vi "classes array.vi"() -> (0 "MBs":refnum<class "Master CR.lvclass">[](array[class]))   [LabVIEW 2021, in "Master CR.lvclass"]
uses:
  Master CR.lvclass
  Devices/M7000/ICPCON PM-3112 RTU/ICPCON PM-3112-RTU.lvclass
  D:/my_projects/projects/Algorithms/Labview/21/Master CR/Master CR.lvclass
  Devices/ET7000/ICPCON ET-7017/ICPCON ET-7017.lvclass
  Devices/ET7000/ICPCON PM-3112/ICPCON PM-3112.lvclass
  Devices/ET7000/ICPCON ET-7051/ICPCON ET-7051.lvclass
  Devices/ET7000/ICPCON ET-7042/ICPCON ET-7042.lvclass
  Devices/ET7000/ICPCON ET-7028/ICPCON ET-7028.lvclass
  Devices/ET7000/ICPCON ET-7024/ICPCON ET-7024.lvclass
  Devices/ET7000/ICPCON ET-7018/ICPCON ET-7018.lvclass
  Devices/ET7000/ICPCON ET-7018i/ICPCON ET-7018i.lvclass
  Devices/ET7000/ICPCON ET-7017-10/ICPCON ET-7017-10.lvclass
  Devices/SMSD/SMSD-DI/SMSD-DI.lvclass
  Devices/SMSD/SMSD-AI/SMSD-AI.lvclass
  Devices/M7000/ICPCON M-7024/ICPCON M-7024.lvclass
  Devices/Serial/ELAN/ELAN.lvclass
  Devices/ET7000/TEST1/TEST1.lvclass
  Devices/ET7000/TEST/TEST.lvclass
  Devices/ET7000/ICPCON ET-7016i/ICPCON ET-7016i.lvclass
  Master CR.lvclass/Master CR.ctl
  Devices/ET7000/ICPCON ET-7042UR/ICPCON ET-7042UR.lvclass
  D:/my_projects/projects/Algorithms/Labview/21/Master CR/Devices/ET7000/TCP/TCP.lvclass
  D:/my_projects/projects/Algorithms/Labview/21/Master CR/Devices/ET7000/TEST/TEST.lvclass
  D:/my_projects/projects/Algorithms/Labview/21/Master CR/Devices/ET7000/TEST1/TEST1.lvclass
  D:/my_projects/projects/Algorithms/Labview/21/Master CR/Devices/ET7000/ICPCON ET-7016i/ICPCON ET-7016i.lvclass
  D:/my_projects/projects/Algorithms/Labview/21/Master CR/Devices/ET7000/ICPCON ET-7017/ICPCON ET-7017.lvclass
  D:/my_projects/projects/Algorithms/Labview/21/Master CR/Devices/ET7000/ICPCON ET-7017-10/ICPCON ET-7017-10.lvclass
  D:/my_projects/projects/Algorithms/Labview/21/Master CR/Devices/ET7000/ICPCON ET-7018i/ICPCON ET-7018i.lvclass
  D:/my_projects/projects/Algorithms/Labview/21/Master CR/Devices/ET7000/ICPCON ET-7018/ICPCON ET-7018.lvclass
  D:/my_projects/projects/Algorithms/Labview/21/Master CR/Devices/ET7000/ICPCON ET-7024/ICPCON ET-7024.lvclass
  D:/my_projects/projects/Algorithms/Labview/21/Master CR/Devices/ET7000/ICPCON ET-7028/ICPCON ET-7028.lvclass
  D:/my_projects/projects/Algorithms/Labview/21/Master CR/Devices/ET7000/ICPCON ET-7042/ICPCON ET-7042.lvclass
  D:/my_projects/projects/Algorithms/Labview/21/Master CR/Devices/ET7000/ICPCON ET-7042UR/ICPCON ET-7042UR.lvclass
  D:/my_projects/projects/Algorithms/Labview/21/Master CR/Devices/ET7000/ICPCON ET-7051/ICPCON ET-7051.lvclass
  D:/my_projects/projects/Algorithms/Labview/21/Master CR/Devices/ET7000/ICPCON PM-3112/ICPCON PM-3112.lvclass
  D:/my_projects/projects/Algorithms/Labview/21/Master CR/Devices/Serial/Modbus Serial/Modbus Serial.lvclass
  D:/my_projects/projects/Algorithms/Labview/21/Master CR/Devices/Serial/Serial.lvclass
  D:/my_projects/projects/Algorithms/Labview/21/Master CR/Devices/M7000/ICPCON M-7024/ICPCON M-7024.lvclass
  D:/my_projects/projects/Algorithms/Labview/21/Master CR/Devices/M7000/ICPCON PM-3112 RTU/ICPCON PM-3112-RTU.lvclass
  D:/my_projects/projects/Algorithms/Labview/21/Master CR/Devices/Serial/ELAN/ELAN.lvclass
  D:/my_projects/projects/Algorithms/Labview/21/Master CR/Devices/SMSD/SMSD.lvclass
  D:/my_projects/projects/Algorithms/Labview/21/Master CR/Devices/SMSD/SMSD-AI/SMSD-AI.lvclass
  D:/my_projects/projects/Algorithms/Labview/21/Master CR/Devices/SMSD/SMSD-DI/SMSD-DI.lvclass
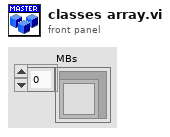
[diagram p1: front panel]
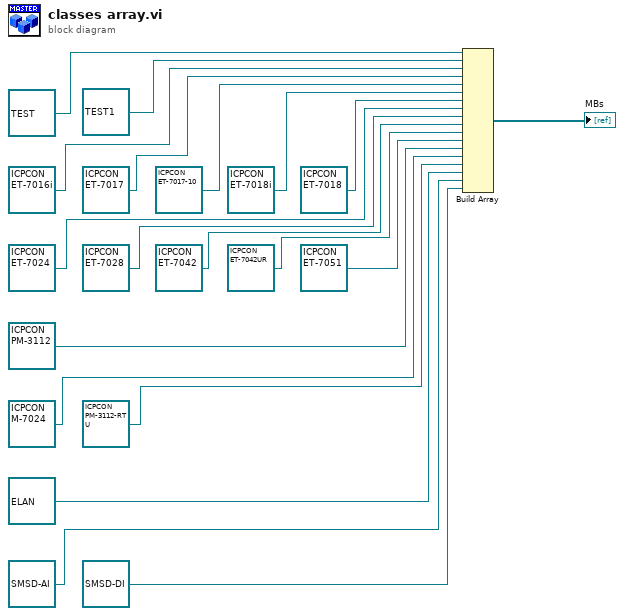
[diagram p0: block diagram]
diagram:
  n1 = Build Array(refnum<class "TEST.lvclass"> refnum ("TEST.lvclass"), refnum<class "TEST1.lvclass"> refnum ("TEST1.lvclass"), refnum<class "ICPCON ET-7016i.lvclass"> refnum ("ICPCON ET-7016i.lvclass"), refnum<class "ICPCON ET-7017.lvclass"> refnum ("ICPCON ET-7017.lvclass"), refnum<class "ICPCON ET-7017-10.lvclass"> refnum ("ICPCON ET-7017-10.lvclass"), refnum<class "ICPCON ET-7018i.lvclass"> refnum ("ICPCON ET-7018i.lvclass"), refnum<class "ICPCON ET-7018.lvclass"> refnum ("ICPCON ET-7018.lvclass"), refnum<class "ICPCON ET-7024.lvclass"> refnum ("ICPCON ET-7024.lvclass"), refnum<class "ICPCON ET-7028.lvclass"> refnum ("ICPCON ET-7028.lvclass"), refnum<class "ICPCON ET-7042.lvclass"> refnum ("ICPCON ET-7042.lvclass"), refnum<class "ICPCON ET-7042UR.lvclass"> refnum ("ICPCON ET-7042UR.lvclass"), refnum<class "ICPCON ET-7051.lvclass"> refnum ("ICPCON ET-7051.lvclass"), refnum<class "ICPCON PM-3112.lvclass"> refnum ("ICPCON PM-3112.lvclass"), refnum<class "ICPCON M-7024.lvclass"> refnum ("ICPCON M-7024.lvclass"), refnum<class "ICPCON PM-3112-RTU.lvclass"> refnum ("ICPCON PM-3112-RTU.lvclass"), refnum<class "ELAN.lvclass"> refnum ("ELAN.lvclass"), refnum<class "SMSD-AI.lvclass"> refnum ("SMSD-AI.lvclass"), refnum<class "SMSD-DI.lvclass"> refnum ("SMSD-DI.lvclass")) -> (→"MBs":refnum<class "Master CR.lvclass">[])
